vi "20170502127惠雨2.vi"() -> ()   [LabVIEW 2017]
panel:
  out "波形图":dbl[](graph)
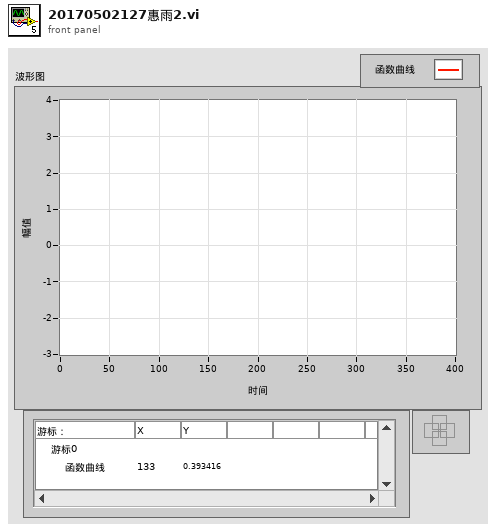
[diagram p1: front panel]
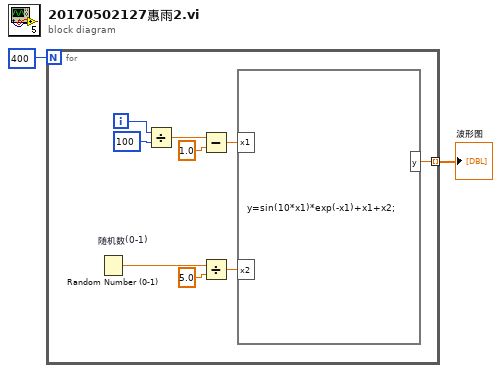
[diagram p0: block diagram]
diagram:
  n1 = for {
    N: 400 -> [_]
    tunnel: [w3] -> w1 mode=indexing
    i -> [w11]
    n2 = Random Number (0-1) "随机数(0-1)"() -> (number: 0 to 1=w7:dbl)
    n3 = Divide(x=w11, y=100) -> (x/y=w9:dbl)
    n4 = Subtract(x=w9, y=1.0) -> (x-y=w5:dbl)
    n5 = Divide(x=w7, y=5.0) -> (x/y=w4:dbl)
    n6 = formula code="y=sin(10*x1)*exp(-x1)+x1+x2;"("x1"=w5, "x2"=w4) -> ("y"=w3:dbl)
  }
  "波形图" <- w1
